vi "CheckFileConformity.vi"(8 "error in (no error)":errorcluster, 10 "File Data":T1, 11 "Path In":path) -> (0 "error out":errorcluster, 2 "No File":bool, 3 "Path Out":path, 5 "Asked to Change?":bool)   [LabVIEW 2019]
uses:
  <userlib>/_OpenG.lib/file/file.llb/Valid Path - Traditional__ogtk.vi
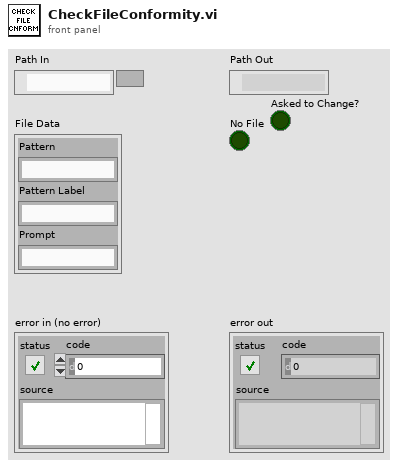
[diagram p1: front panel]
types:
  T1 = cluster{"Pattern":string, "Pattern Label":string, "Prompt":string}
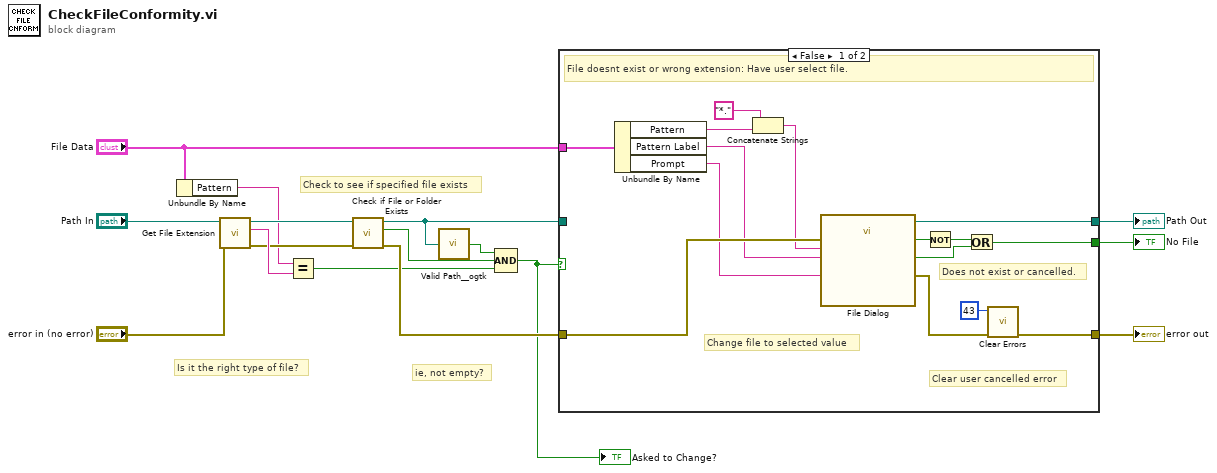
[diagram p0: block diagram]
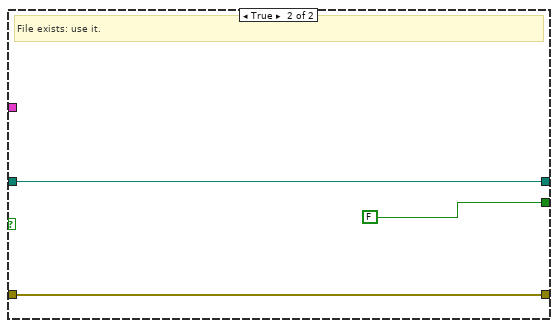
[diagram p2: hidden frame]
diagram:
  # "ie, not empty?"
  # "Is it the right type of file?"
  # "Check to see if specified file exists"
  n1 = Unbundle By Name("File Data") -> ("Pattern"=w6:string)
  n2 = call <vilib>:"Get File Extension.vi"("error in (no error)"="error in (no error)", "file"="Path In") -> ("error out"=w14:errorcluster, "lowercase file extension"=w16:string, "dup file"=w15:path)  [unwired: 5 in, 2 out]
  n3 = Equal?(x=w6, y=w16) -> (x = y?=w11:bool)
  n4 = call <vilib>:"Check if File or Folder Exists.vi"("error in (no error)"=w14, "path"=w15) -> ("error out"=w13:errorcluster, "file or folder exists?"=w12:bool, "dup path"=w1:path)  [unwired: 7 in]
  n5 = call-poly <userlib>:"Valid Path__ogtk.vi"("path"=w1) -> ("valid"=w2:bool)
  n6 = Compound Arithmetic op=AND(w2, w12, w11) -> (w10:bool)
  "Asked to Change?" <- w10
  n7 = case shown="False" w10 {
    tunnel: w1 -> [_ w33]
    tunnel: w13 -> [w31 w34]
    tunnel: [w29 w33] -> w7
    tunnel: [w18 w34] -> w8
    tunnel: "File Data" -> [w28 _]
    tunnel: [w19 FALSE ("cancelled")] -> w4
    frame False {
      # "Clear user cancelled error"
      # "Does not exist or cancelled."
      # "Change file to selected value"
      # "File doesnt exist or wrong extension: Have user select file."
      n8 = Unbundle By Name(w28) -> ("Pattern"=w27:string, "Pattern Label"=w25:string, "Prompt"=w24:string)
      n9 = Concatenate Strings("*." ("string"), w27) -> (w26:string)
      n10 = call "File Dialog"("prompt"=w24, "error in"=w31, "pattern (all files)"=w26, "pattern label"=w25) -> ("selected path"=w29:path, "exists"=w22:bool, "cancelled"=w20:bool, "error out"=w30:errorcluster)  [unwired: 8 in]
      n11 = Not(x=w22) -> (.not. x?=w21:bool)
      n12 = Or(x=w21, y=w20) -> (x .or. y?=w19:bool)
      n13 = call <vilib>:"Clear Errors.vi"("error in (no error)"=w30, "specific error code to clear (0: all)"=43) -> ("error out"=w18:errorcluster)  [unwired: 4 in, 1 out]
    }
    frame True {
      # "File exists: use it."
    }
  }
  "Path Out" <- w7
  "error out" <- w8
  "No File" <- w4
